vi "원격실행.vi"() -> ()   [LabVIEW 2014]
panel:
  in  "vi 경로":path
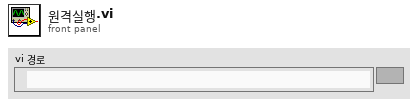
[diagram p1: front panel]
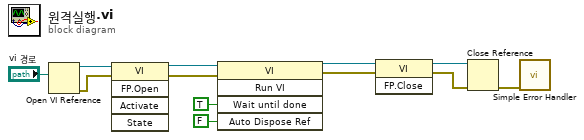
[diagram p0: block diagram]
diagram:
  n1 = Open VI Reference(vi path="vi 경로") -> (vi reference=w11:refnum<vi>, error out=w10:errorcluster)  [unwired: 5 in]
  n2 = invoke class="VI" method="FP.Open"(reference=w11, error in=w10) -> (reference out=w9:refnum<vi>, error out=w8:errorcluster)  [unwired: 3 in, 3 out]
  n3 = invoke class="VI" method="Run VI"(reference=w9, error in=w8, "Wait until done"=TRUE ("완료될 때까지 기다림"), "Auto Dispose Ref"=FALSE ("참조 자동 삭제")) -> (reference out=w5:refnum<vi>, error out=w4:errorcluster)  [unwired: 1 in, 3 out]
  n4 = invoke class="VI" method="FP.Close"(reference=w5, error in=w4) -> (reference out=w3:refnum<vi>, error out=w2:errorcluster)  [unwired: 1 in, 1 out]
  n5 = Close Reference(reference=w3, error in (no error)=w2) -> (error out=w1:errorcluster)
  n6 = call <vilib>:"Simple Error Handler.vi"("error in (no error)"=w1) -> ()  [unwired: 4 in, 5 out]
